vi "Toggle.vi"(7 "Initial Value":bool, 11 "In":bool) -> (3 "Toggled":bool)   [LabVIEW 2014]
uses:
  Change Detect Boolean.vi
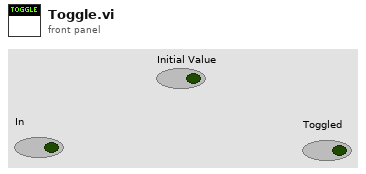
[diagram p1: front panel]
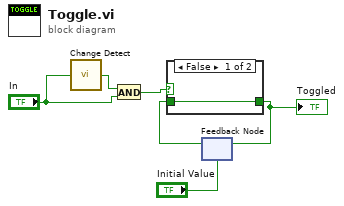
[diagram p0: block diagram]
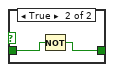
[diagram p2: hidden frame]
diagram:
  n1 = call-poly "Change Detect.vi"("In"="In") -> ("Changed?"=w5:bool)
  n2 = And(x=w5, y="In") -> (x .and. y?=w3:bool)
  n3 = feedback #1("Initial Value") -> (w2:bool)
  n4 = case shown="False" w3 {
    tunnel: w2 -> [w7 w8]
    tunnel: [w7 w9] -> w1
    frame False {
    }
    frame True {
      n5 = Not(x=w8) -> (.not. x?=w9:bool)
    }
  }
  "Toggled" <- w1
  n6 = feedback-in #1(w1) -> ()
